vi "PXI-Flush AI Queue.vi"(11 "error in (no error)":errorcluster) -> (15 "error out":errorcluster)   [LabVIEW 2020]
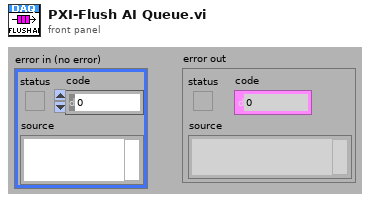
[diagram p1: front panel]
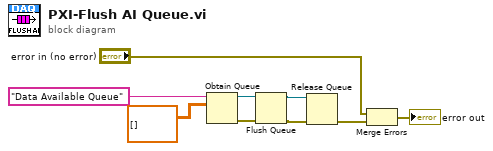
[diagram p0: block diagram]
diagram:
  n1 = Obtain Queue(name (unnamed)="Data Available Queue", element data type=dbl[][] [] ("AI Waveforms 2")) -> (queue out=w1:refnum<queue>, error out=w6:errorcluster)  [unwired: 3 in, 1 out]
  n2 = Flush Queue(queue=w1, error in (no error)=w6) -> (queue out=w4:refnum<queue>, error out=w5:errorcluster)  [unwired: 1 out]
  n3 = Release Queue(queue=w4, error in (no error)=w5) -> (error out=w9:errorcluster)  [unwired: 1 in, 2 out]
  n4 = Merge Errors("error in (no error)", w9) -> (→"error out":errorcluster)
